vi "Resetting Drive Encoders.vi"(1 "Reset Encoders":bool) -> ()   [LabVIEW 2014]
uses:
  Begin/Global RefNums.vi
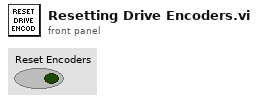
[diagram p1: front panel]
types:
  T1 = typedef "WPI_CounterDevRef.ctl" = cluster{"DevStatus":errorcluster, "CntIndex":T2}
  T2 = typedef "FPGA_CounterCtrSystemIndex.ctl" = enum8{"Ctr 0", "Ctr 1", "Ctr 2", "Ctr 3", "Ctr 4", "Ctr 5", "Ctr 6", "Ctr 7", "Invalid"}
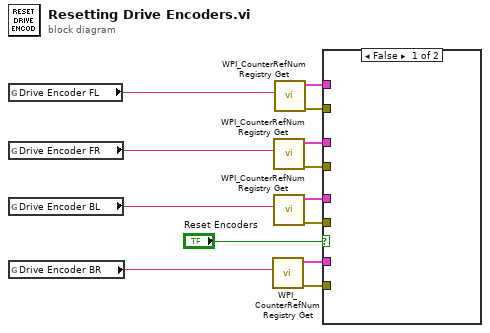
[diagram p0: block diagram]
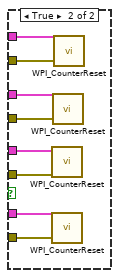
[diagram p2: hidden frame]
diagram:
  n1 = global read "Global RefNums.vi" "Drive Encoder FL"() -> (w4:string)
  n2 = global read "Global RefNums.vi" "Drive Encoder FR"() -> (w3:string)
  n3 = global read "Global RefNums.vi" "Drive Encoder BL"() -> (w2:string)
  n4 = global read "Global RefNums.vi" "Drive Encoder BR"() -> (w1:string)
  n5 = call <vilib>:"WPI_CounterRefNum Registry Get.vi"("refnum name"=w1) -> ("error out"=w6:errorcluster, "CounterDevRef"=w7:T1)  [unwired: 9 in]
  n6 = call <vilib>:"WPI_CounterRefNum Registry Get.vi"("refnum name"=w3) -> ("error out"=w10:errorcluster, "CounterDevRef"=w11:T1)  [unwired: 9 in]
  n7 = call <vilib>:"WPI_CounterRefNum Registry Get.vi"("refnum name"=w2) -> ("error out"=w8:errorcluster, "CounterDevRef"=w9:T1)  [unwired: 9 in]
  n8 = call <vilib>:"WPI_CounterRefNum Registry Get.vi"("refnum name"=w4) -> ("error out"=w12:errorcluster, "CounterDevRef"=w13:T1)  [unwired: 9 in]
  n9 = case shown="False" "Reset Encoders" {
    tunnel: w13 -> [_ w21]
    tunnel: w12 -> [_ w20]
    tunnel: w11 -> [_ w19]
    tunnel: w10 -> [_ w18]
    tunnel: w9 -> [_ w17]
    tunnel: w8 -> [_ w16]
    tunnel: w7 -> [_ w15]
    tunnel: w6 -> [_ w14]
    frame False {
    }
    frame True {
      n10 = call <vilib>:"WPI_CounterReset.vi"("error in (no error)"=w16, "CounterDevRef in"=w17) -> ()  [unwired: 8 in, 2 out]
      n11 = call <vilib>:"WPI_CounterReset.vi"("error in (no error)"=w14, "CounterDevRef in"=w15) -> ()  [unwired: 8 in, 2 out]
      n12 = call <vilib>:"WPI_CounterReset.vi"("error in (no error)"=w18, "CounterDevRef in"=w19) -> ()  [unwired: 8 in, 2 out]
      n13 = call <vilib>:"WPI_CounterReset.vi"("error in (no error)"=w20, "CounterDevRef in"=w21) -> ()  [unwired: 8 in, 2 out]
    }
  }
